vi "Waveform_Read Write End Point Index.vi"(6 "Read(f)\nWrite(t)":T1, 8 "Error":errorcluster, 10 "End Point":i32, 11 "Waveform Atributes":variant) -> (0 "Error Out":errorcluster, 2 "End Point Out":i32, 3 "Waveform Atributes Out":variant)   [LabVIEW 2016]
uses:
  Universal Controls/Read Write Button.ctl
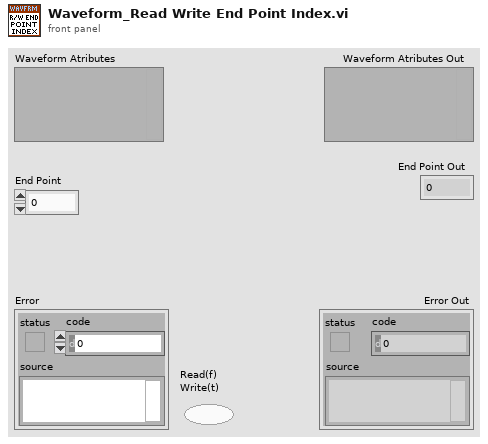
[diagram p1: front panel]
types:
  T1 = typedef "Read Write Button.ctl" = bool
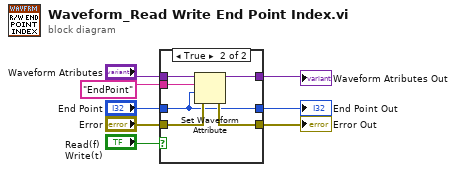
[diagram p0: block diagram]
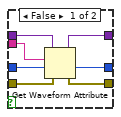
[diagram p2: hidden frame]
diagram:
  n1 = case shown="True" "Read(f)\nWrite(t)" {
    tunnel: [w15 w17] -> w8
    tunnel: "Waveform Atributes" -> [w14 w18]
    tunnel: "End Point" -> [w13 w16]
    tunnel: "EndPoint" ("name") -> [w12 w21]
    tunnel: "Error" -> [w11 w20]
    tunnel: [w10 w19] -> w3
    tunnel: [w9 w16] -> w2
    frame False {
      n2 = Get Waveform Attribute(4:w11, 5:w13, 6:w12, 7:w14) -> (0:w10:errorcluster, 1:w9:i32, 3:w15:variant)  [unwired: 1 out]
    }
    frame True {
      n3 = Set Waveform Attribute(4:w20, 5:w16, 6:w21, 7:w18) -> (0:w19:errorcluster, 3:w17:variant)  [unwired: 1 out]
    }
  }
  "Waveform Atributes Out" <- w8
  "Error Out" <- w3
  "End Point Out" <- w2
